vi "S1500_S7Com_from_PLC(SubVI).vi"(3 "S7Com_Data_Array_In":T2) -> (1 "from_PLC_Out":T1)   [LabVIEW 2018]
doc: "Distributes the PLC data into the Labview cluster."
uses:
  S7Com_Source_inkl_IP/S7Com_Data_Array.ctl
  S1500_S7Com_PLC_Data.ctl
panel:
  # "This subVI unpacks the PLC data array into the data cluster."
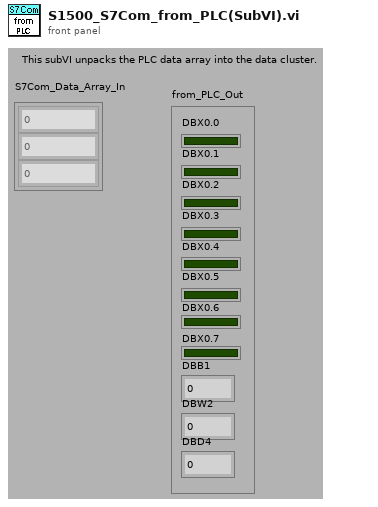
[diagram p1: front panel]
types:
  T1 = typedef "S1500_S7Com_PLC_Data.ctl" = cluster{"DBX0.0":bool, "DBX0.1":bool, "DBX0.2":bool, "DBX0.3":bool, "DBX0.4":bool, "DBX0.5":bool, "DBX0.6":bool, "DBX0.7":bool, "DBB1":i8, "DBW2":i16, "DBD4":i32}
  T2 = typedef "S7Com_Data_Array.ctl" = i32[]
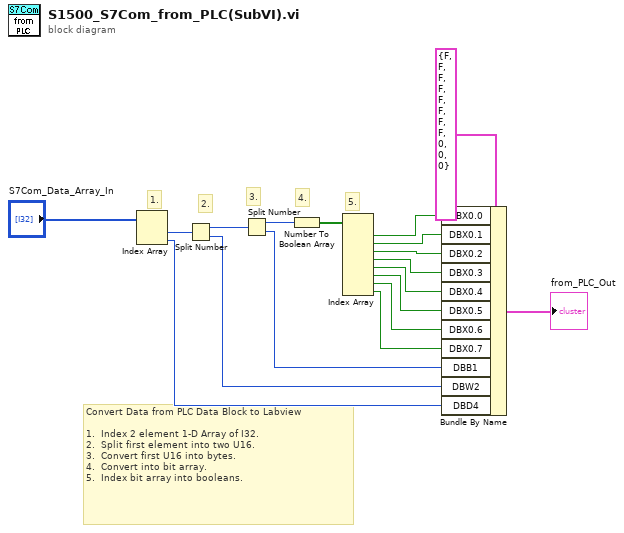
[diagram p0: block diagram]
diagram:
  # "Convert Data from PLC Data Block to Labview\n\n1.  Index 2 element 1-D Array of I32.\n2.  Split first element into two U16.\n3.  Convert first U16 into bytes.\n4.  Convert into bit array.\n5.  Index bit array into booleans."
  # "5."
  # "4."
  # "3."
  # "2."
  # "1."
  n1 = Index Array(array="S7Com_Data_Array_In") -> (element #1=w17:i32, element #2=w11:i32)  [unwired: 2 in]
  n2 = Split Number(x=w17) -> (hi(x)=w16:u16, lo(x)=w12:u16)
  n3 = Split Number(x=w16) -> (hi(x)=w10:u8, lo(x)=w13:u8)
  n4 = Number To Boolean Array(number=w10) -> (Boolean array=w9:bool[])
  n5 = Index Array(array=w9) -> (element #1=w8:bool, element #2=w7:bool, element #3=w6:bool, element #4=w5:bool, element #5=w4:bool, element #6=w3:bool, element #7=w2:bool, element #8=w1:bool)  [unwired: 8 in]
  n6 = Bundle By Name(cluster=T1 {"DBX0.0"=FALSE, "DBX0.1"=FALSE, "DBX0.2"=FALSE, "DBX0.3"=FALSE, "DBX0.4"=FALSE, "DBX0.5"=FALSE, "DBX0.6"=FALSE, "DBX0.7"=FALSE, "DBB1"=0, "DBW2"=0, "DBD4"=0} ("PLC"), "DBX0.0"=w8, "DBX0.1"=w7, "DBX0.2"=w6, "DBX0.3"=w5, "DBX0.4"=w4, "DBX0.5"=w3, "DBX0.6"=w2, "DBX0.7"=w1, "DBB1"=w13, "DBW2"=w12, "DBD4"=w11) -> (→"from_PLC_Out":T1)
